vi "Begin.vi"() -> (1 "Образец № 2":string)   [LabVIEW 2018]
panel:
  in  "Образец №":string
  in  "Ввел!":bool
  out "Boolean":bool
  out "Boolean 2":bool
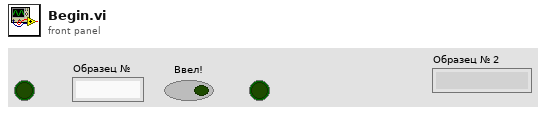
[diagram p1: front panel]
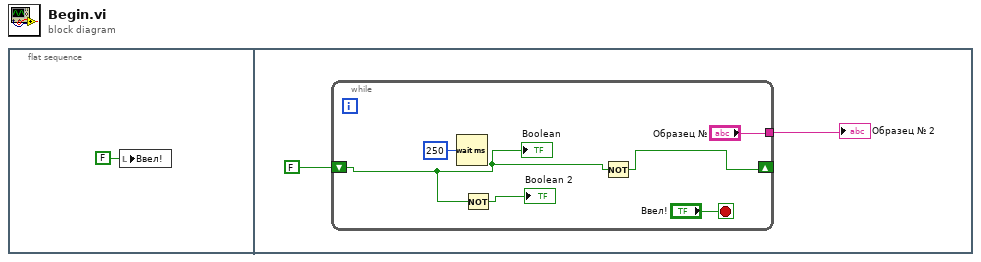
[diagram p0: block diagram]
diagram:
  n1 = flat-sequence {
    frame #0 {
      n2 = local write "Ввел!"(FALSE ("Ввел!")) -> ()
    }
    frame #1 {
      n3 = while {
        tunnel: ["Образец №"] -> w3
        shift-right: [w4] -> _
        shift-left: FALSE -> [w5]
        stop <- "Ввел!" stop-if-true
        n4 = Wait (ms)(milliseconds to wait=u32 250) -> ()  [unwired: 1 out]
        n5 = Not(x=w5) -> (.not. x?=→"Boolean 2":bool)
        n6 = Not(x=w5) -> (.not. x?=w4:bool)
        "Boolean" <- w5
      }
      "Образец № 2" <- w3
    }
  }
